vi "DSP.GetEvents.vi"(8 "error in (no error)":errorcluster, 11 "DSP in":refnum<class "DSP.lvclass">) -> (0 "error out":errorcluster, 3 "DSP":cluster{"Public Events":T1, "Public Events":T2})   [LabVIEW 2016, in "DSP.lvclass"]
uses:
  DSP.lvclass
  <vilib>/JKI/JKI SMO/SMO/Typedefs/Public Events.ctl
  <vilib>/JKI/JKI SMO/SMO/Typedefs/SMOState --Enum.ctl
  <vilib>/JKI/JKI SMO/SMO/Typedefs/Reserve State--Enum.ctl
  Typedefs/PublicEvents--Cluster.ctl
  Typedefs/PublicEvents--DSP.getWaveforms.ctl
  Typedefs/PublicEvents--DSP.getLockin.ctl
  DSP.lockin/Typedefs/LockinResult.ctl
  Typedefs/PublicEvents--DSP.getPowerSpectrum.ctl
  C:/Program Files (x86)/National Instruments/LabVIEW 2016/vi.lib/JKI/JKI SMO/SMO/SMO.lvclass
  <vilib>/JKI/JKI SMO/SMO/SMO.lvclass
  DSP.lockin/DSP_lockin.lvclass
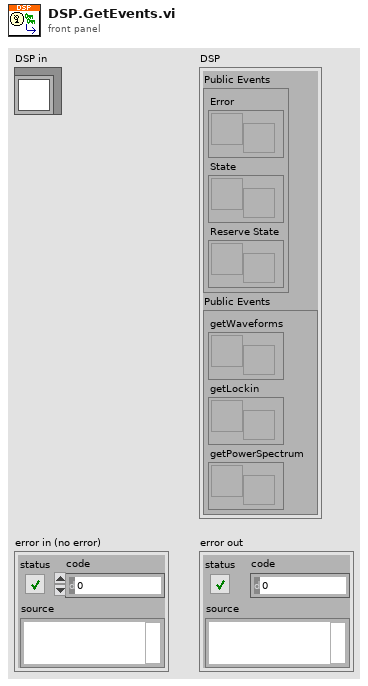
[diagram p1: front panel]
types:
  T1 = typedef "SMO.lvclass/Public Events.ctl" = cluster{"Error":refnum<user-event>, "State":refnum<user-event>, "Reserve State":refnum<user-event>}
  T2 = typedef "DSP.lvclass/PublicEvents--Cluster.ctl" = cluster{"getWaveforms":refnum<user-event>, "getLockin":refnum<user-event>, "getPowerSpectrum":refnum<user-event>}
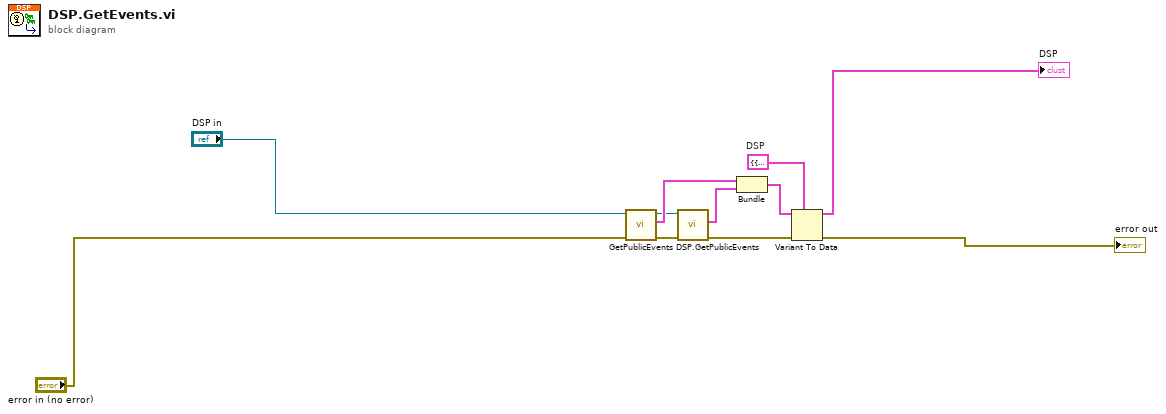
[diagram p0: block diagram]
diagram:
  w8 = cluster{"Public Events":T1, "Public Events":T2} {"Public Events"={"Error"=refnum, "State"=refnum, "Reserve State"=refnum}, "Public Events"={"getWaveforms"=refnum, "getLockin"=refnum, "getPowerSpectrum"=refnum}}  # DSP
  n1 = call <vilib>:"GetPublicEvents.vi"("error in (no error)"="error in (no error)", "SMO"="DSP in") -> ("error out"=w5:errorcluster, "Public Events"=w3:T1, "SMO out"=w1:refnum<class "DSP.lvclass">)  [unwired: 7 in]
  n2 = call "DSP.GetPublicEvents.vi"("error in (no error)"=w5, "DSP"=w1) -> ("error out"=w9:errorcluster, "Public Events"=w4:T2)  [unwired: 7 in, 1 out]
  n3 = Bundle("Public Events"=w3, "Public Events"=w4) -> (w6:cluster{"Public Events":T1, "Public Events":T2})  [unwired: 1 in]
  n4 = Variant To Data(error in=w9, type=w8, Variant=w6) -> (data=→"DSP":cluster{"Public Events":T1, "Public Events":T2}, error out=→"error out":errorcluster)
